vi "Grab Hatch Panel in Auto.vi"   [LabVIEW 2018]
uses:
  SubSystems/Hatch Panel Intake/Hatch Panel Intake Global.vi
  SubSystems/Cargo Intake/Cargo Intake Global.vi
  SubSystems/Lift/Lift Global.vi
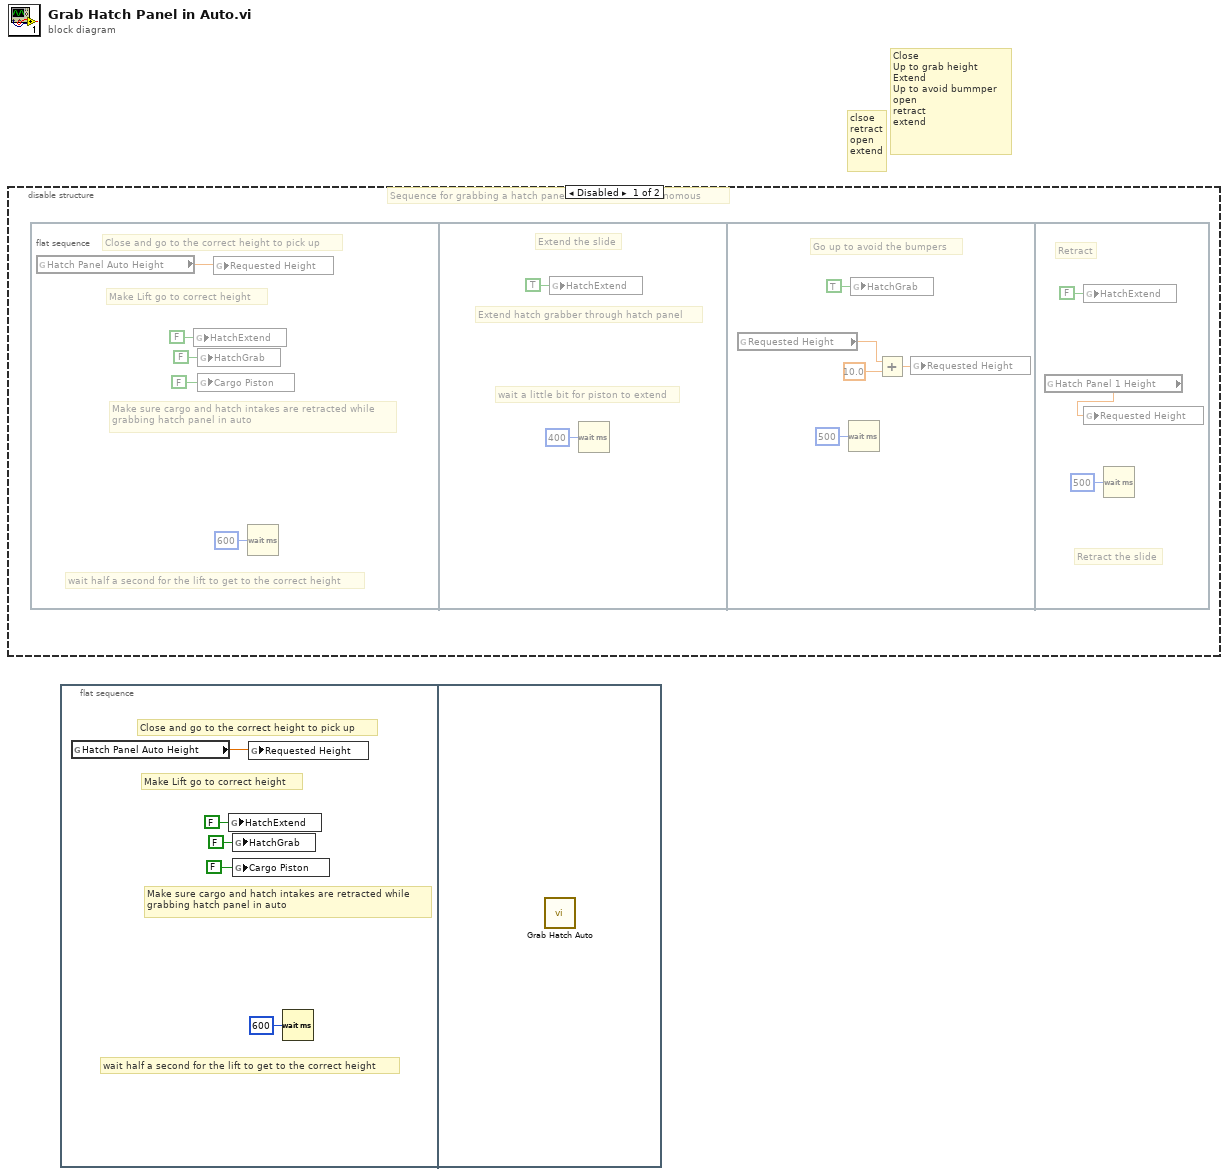
[diagram p0: block diagram]
diagram:
  # "clsoe\nretract\nopen\nextend"
  # "Close\nUp to grab height\nExtend\nUp to avoid bummper\nopen\nretract\nextend"
  n1 = disable-structure shown="Disabled" {
    frame Disabled {
      # "Sequence for grabbing a hatch panel at the start of autonomous"
      n2 = flat-sequence {
        frame #0 {
          # "Close and go to the correct height to pick up"
          # "Make sure cargo and hatch intakes are retracted while\ngrabbing hatch panel in auto"
          # "wait half a second for the lift to get to the correct height"
          # "Make Lift go to correct height"
          n3 = global read "Lift Global.vi" "Hatch Panel Auto Height"() -> (w5:dbl)
          n4 = global write "Hatch Panel Intake Global.vi" "HatchExtend"(FALSE ("HatchExtend")) -> ()
          n5 = global write "Hatch Panel Intake Global.vi" "HatchGrab"(FALSE ("HatchGrab")) -> ()
          n6 = global write "Cargo Intake Global.vi" "Cargo Piston"(FALSE ("Cargo Piston")) -> ()
          n7 = global write "Lift Global.vi" "Requested Height"(w5) -> ()
          n8 = Wait (ms)(milliseconds to wait=u32 600) -> ()  [unwired: 1 out]
        }
        frame #1 {
          # "Extend the slide"
          # "wait a little bit for piston to extend"
          # "Extend hatch grabber through hatch panel"
          n9 = global write "Hatch Panel Intake Global.vi" "HatchExtend"(TRUE ("HatchExtend")) -> ()
          n10 = Wait (ms)(milliseconds to wait=u32 400) -> ()  [unwired: 1 out]
        }
        frame #2 {
          # "Go up to avoid the bumpers"
          n11 = global read "Lift Global.vi" "Requested Height"() -> (w10:dbl)
          n12 = Wait (ms)(milliseconds to wait=u32 500) -> ()  [unwired: 1 out]
          n13 = global write "Hatch Panel Intake Global.vi" "HatchGrab"(TRUE ("HatchGrab")) -> ()
          n14 = Add(x=w10, y=10.0) -> (x+y=w11:dbl)
          n15 = global write "Lift Global.vi" "Requested Height"(w11) -> ()
        }
        frame #3 {
          # "Retract"
          # "Retract the slide"
          n16 = global read "Lift Global.vi" "Hatch Panel 1 Height"() -> (w13:dbl)
          n17 = global write "Hatch Panel Intake Global.vi" "HatchExtend"(FALSE ("HatchExtend")) -> ()
          n18 = global write "Lift Global.vi" "Requested Height"(w13) -> ()
          n19 = Wait (ms)(milliseconds to wait=u32 500) -> ()  [unwired: 1 out]
        }
      }
    }
    frame Enabled {
    }
  }
  n20 = flat-sequence {
    frame #0 {
      # "Close and go to the correct height to pick up"
      # "Make sure cargo and hatch intakes are retracted while\ngrabbing hatch panel in auto"
      # "wait half a second for the lift to get to the correct height"
      # "Make Lift go to correct height"
      n21 = global read "Lift Global.vi" "Hatch Panel Auto Height"() -> (w20:dbl)
      n22 = global write "Hatch Panel Intake Global.vi" "HatchExtend"(FALSE ("HatchExtend")) -> ()
      n23 = global write "Hatch Panel Intake Global.vi" "HatchGrab"(FALSE ("HatchGrab")) -> ()
      n24 = global write "Cargo Intake Global.vi" "Cargo Piston"(FALSE ("Cargo Piston")) -> ()
      n25 = global write "Lift Global.vi" "Requested Height"(w20) -> ()
      n26 = Wait (ms)(milliseconds to wait=u32 600) -> ()  [unwired: 1 out]
    }
    frame #1 {
      n27 = call "Grab Hatch Auto.vi"() -> ()  [unwired: 12 in]
    }
  }
